vi "Test Frame Rate.vi"() -> ()   [LabVIEW 2013]
uses:
  <vilib>/Utility/file.llb/Write To Spreadsheet File (DBL).vi
panel:
  out "Dropped Frames":i32[](graph)
  out "Iteration":i32
  out "Frame Rate":dbl[](graph)
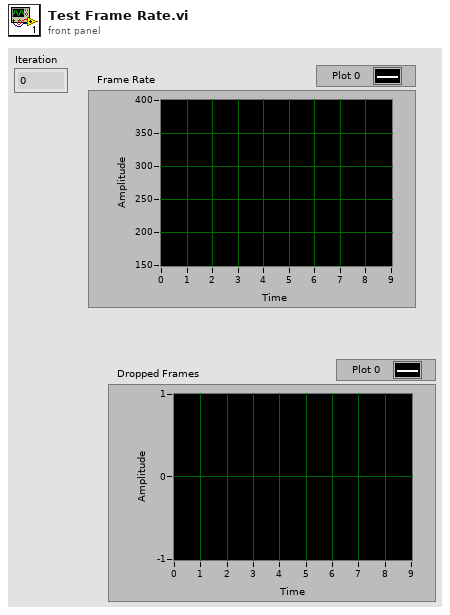
[diagram p1: front panel]
types:
  T1 = cluster{"Horizontal Offset":i32, "Vertical Offset":i32, "Horizontal Width":i32, "Vertical Width":i32}
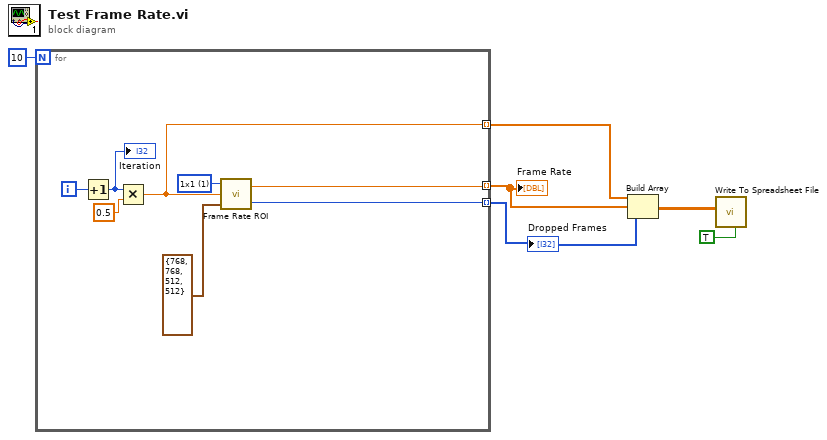
[diagram p0: block diagram]
diagram:
  n1 = for {
    N: 10 -> [_]
    tunnel: [w10] -> w5 mode=indexing
    tunnel: [w9] -> w4 mode=indexing
    tunnel: [w7] -> w2 mode=indexing
    i -> [w12]
    w14 = u16 1 items=["1x1"=1, "2x2"=2, "4x4"=4] ("Binning")
    n2 = Increment(x=w12) -> (x+1=w8:i32)
    "Iteration" <- w8
    n3 = Multiply(x=w8, y=0.5) -> (x*y=w7:dbl)
    n4 = call "Frame Rate ROI.vi"("ROI"=T1 {"Horizontal Offset"=768, "Vertical Offset"=768, "Horizontal Width"=512, "Vertical Width"=512}, "Exposure (ms)"=w7, "Binning"=w14) -> ("Dropped Frames"=w9:i32, "Frame Rate"=w10:dbl)
  }
  "Frame Rate" <- w5
  "Dropped Frames" <- w4
  n5 = Build Array(w2, w5, w4) -> (w3:dbl[][])
  n6 = call-poly <vilib>:"Write To Spreadsheet File.vi"("transpose? (no:F)"=TRUE, "2D data"=w3) -> ()  [unwired: 6 in, 1 out]
